vi "ConfigureAcquisition.vi"(8 "error in (no error)":errorcluster, 11 "NIScope in":refnum<class "NIScope.lvclass">) -> (0 "error out":errorcluster, 3 "NIScope out":refnum<class "NIScope.lvclass">)   [LabVIEW 2018, in "ScopePlugins.lvlib" / "NIScope.lvclass"]
doc: "This VI configures the horizontal settings."
uses:
  NIScope.lvclass
  C:/projects/ICDAS/NistPluggableModules/Scope/ScopePlugins/ScopePluginBaseClass/ScopePluginsBase.lvclass
  ScopePluginBaseClass/ScopePluginsBase.lvclass/ScopePluginsBase.ctl
  NIScope.lvclass/NIScope.ctl
  <instrlib>/niScope/Controls/niScope acquisition type.ctl
  ScopePluginBaseClass/Accessors/Write Channels.vi
  ScopePluginBaseClass/Accessors/Read Channels.vi
  <vilib>/Utility/error.llb/Error Cluster From Error Code.vi
  <vilib>/ErrorRing/Error Ring.xnode
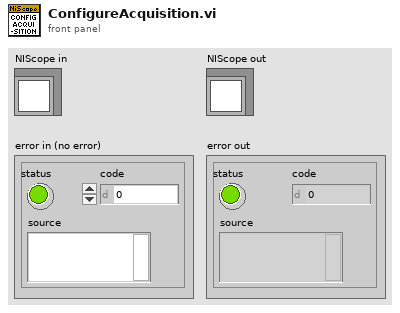
[diagram p1: front panel]
types:
  T1 = typedef "ScopePlugins.lvlib/ScopePluginsBase.lvclass/InitializationSettings.ctl" = cluster{"Reset":bool, "IdQuery":bool, "AutoConfig":bool, "Options String":string, "Synchronize":bool}
  T2 = typedef "ScopePlugins.lvlib/ScopePluginsBase.lvclass/ChannelSetting(s).ctl" = cluster{"Number of Channels":i32, "Channel(s)":cluster{"Enabled":bool, "Instrument Handle":string, "Channel Name":string, "Maximum Input Frequency":dbl, "Verticle Settings":cluster{"Vertical Range":dbl, "Vertical Offset":dbl, "Probe Attenuation":dbl, "Vertical Coupling":i32}, "Connected":bool, "Input Impedance":dbl, "IO Type Instrument Handle":refnum<k15>}[]}
  T3 = cluster{"Enabled":bool, "Instrument Handle":string, "Channel Name":string, "Maximum Input Frequency":dbl, "Verticle Settings":cluster{"Vertical Range":dbl, "Vertical Offset":dbl, "Probe Attenuation":dbl, "Vertical Coupling":i32}, "Connected":bool, "Input Impedance":dbl, "IO Type Instrument Handle":refnum<k15>}[]
  T4 = typedef "ScopePlugins.lvlib/ScopePluginsBase.lvclass/HorizontalSettings.ctl" = cluster{"Continuous":bool, "EnableAveraging":bool, "Number Averages":i32, "Measurement Timeout":dbl, "Min Record Length":i32, "Min Sample Rate":dbl, "Enforce Realtime":bool, "Sampling Mode ":enum16{"Real Time", "Equivalent Time", "Segment", "Real Time Peak Detect", "Real Time High Resolution", "Peak Detect Segment", "High Resolution Segment"}, "Interpolation":enum16{"No Interpolation", "sin(x)/x", "linear", "1 Point sin(x)/x", "2 Point sin(x)/x", "4 Point sin(x)/x", "8 Point sin(x)/x", "16 Point sin(x)/x"}, "Type":enum16{"Normal", "PeakDetect", "HighRes", "Envelope", "Average"}, "StartTime":dbl, "Time Per Record":dbl, "Number of Points Minimum":i32, "Measurement Name":string, "Measurement RefreshTime (ms)":u32}
  T5 = enum16{"Normal", "PeakDetect", "HighRes", "Envelope", "Average"}
  T6 = typedef "niScope acquisition type.ctl" = i32
  T7 = cluster{"Enabled":bool, "Instrument Handle":string, "Channel Name":string, "Maximum Input Frequency":dbl, "Verticle Settings":cluster{"Vertical Range":dbl, "Vertical Offset":dbl, "Probe Attenuation":dbl, "Vertical Coupling":i32}, "Connected":bool, "Input Impedance":dbl, "IO Type Instrument Handle":refnum<k15>}
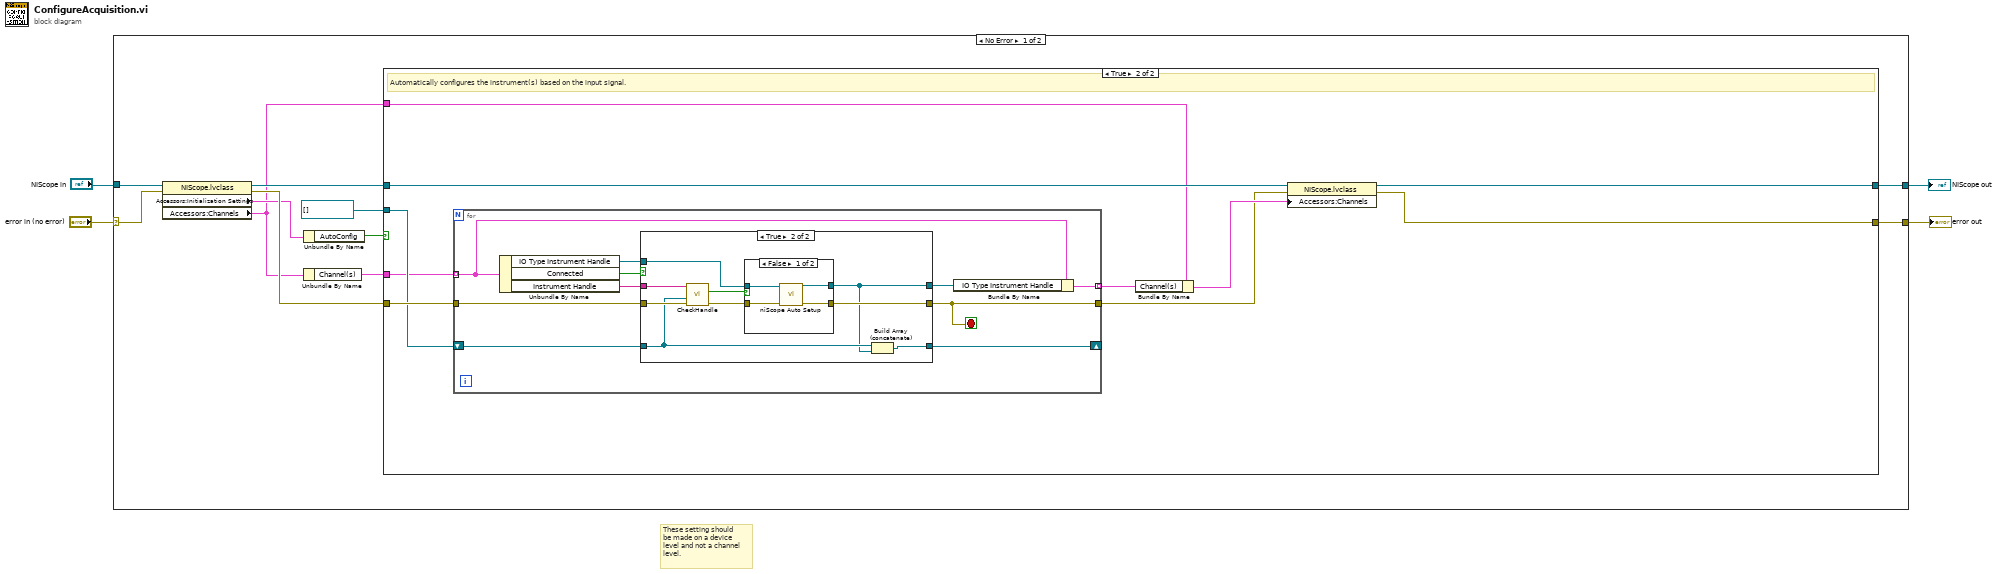
[diagram p0: block diagram]
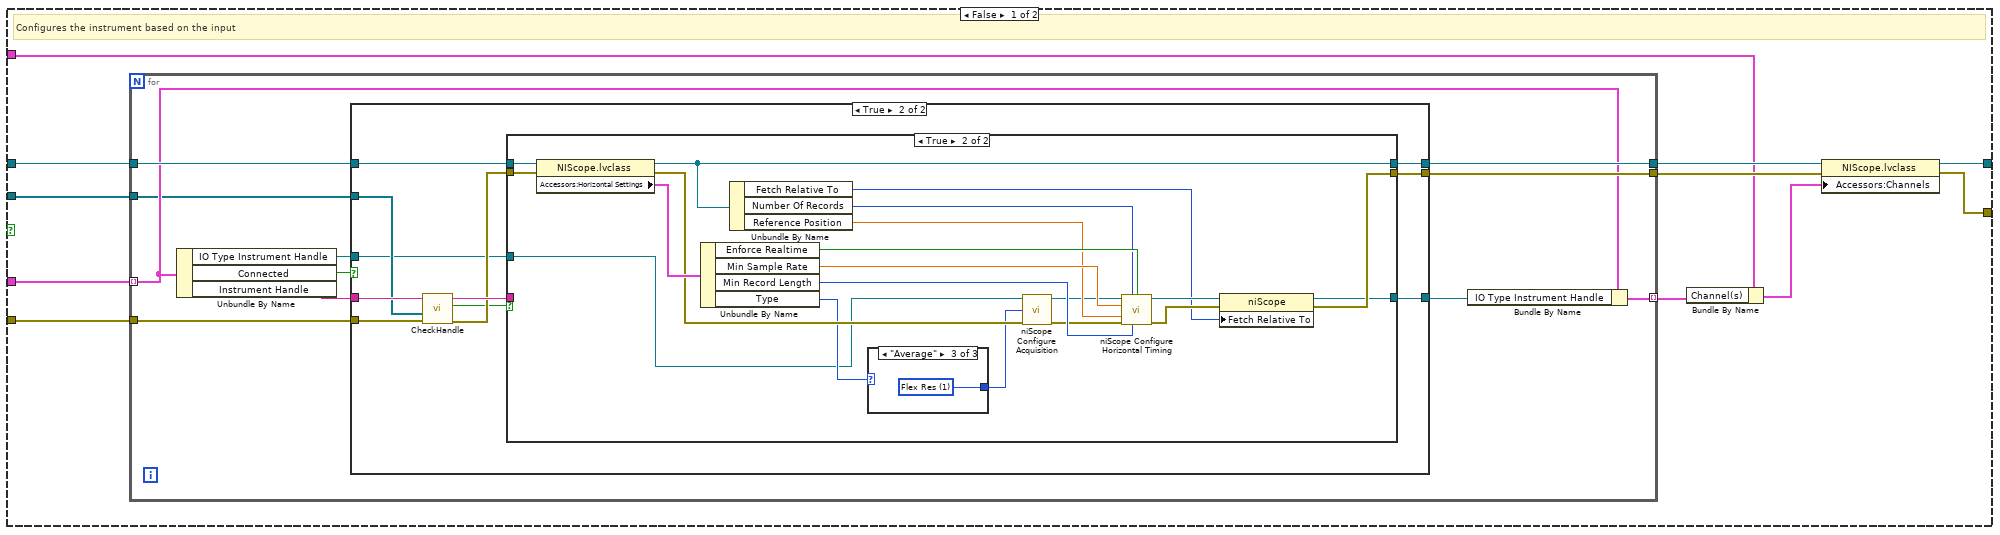
[diagram p2: hidden frame]
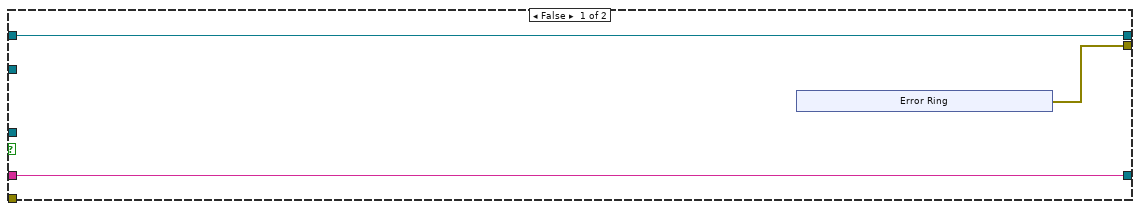
[diagram p3: hidden frame]
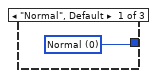
[diagram p5: hidden frame]
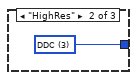
[diagram p6: hidden frame]
diagram:
  # "These setting should\nbe made on a device\nlevel and not a channel\nlevel."
  n1 = case shown="No Error" "error in (no error)" {
    selector: "error in (no error)" -> [w15 w121]
    tunnel: "NIScope in" -> [w14 w122]
    tunnel: [w10 w122] -> w2
    tunnel: [w9 w121] -> w1
    frame No Error {
      n2 = property class="NIScope.lvclass"(reference=w14, error in=w15) -> (reference out=w13:refnum<class "NIScope.lvclass">, error out=w12:errorcluster, "Accessors:Initialization Settings"=w6:T1, "Accessors:Channels"=w5:T2)
      n3 = Unbundle By Name(w6) -> ("AutoConfig"=w8:bool)
      n4 = Unbundle By Name(w5) -> ("Channel(s)"=w11:T3)
      n5 = case shown="True" w8 {
        tunnel: w13 -> [w25 w88]
        tunnel: w12 -> [w24 w92]
        tunnel: w11 -> [w17 w85]
        tunnel: [w23 w89] -> w10
        tunnel: [w21 w87] -> w9
        tunnel: refnum<k15>[] [] ("Array") -> [w18 w91]
        tunnel: w5 -> [w16 w83]
        frame False {
          # "Configures the instrument based on the input"
          n6 = for {
            tunnel: [w37] -> w26
            tunnel: w25 -> [w36]
            tunnel: w17 -> [w30] mode=indexing
            tunnel: [w31] -> w19 mode=indexing
            tunnel: w18 -> [w28]
            tunnel: w24 -> [w35]
            tunnel: [w33] -> w22
            n7 = Unbundle By Name(w30) -> ("IO Type Instrument Handle"=w27:refnum<k15>, "Connected"=w29:bool, "Instrument Handle"=w34:string)
            n8 = case shown="True" w29 {
              tunnel: w36 -> [w40 w56]
              tunnel: [w40 w55] -> w37
              tunnel: [w39 w53] -> w33
              tunnel: w35 -> [_ w49]
              tunnel: w34 -> [w38 w52]
              tunnel: [w38 w54] -> w32
              tunnel: w28 -> [_ w51]
              tunnel: w27 -> [_ w46]
              frame False {
                n9 = xnode "Error Ring"() -> ("error out"=w39:errorcluster)
              }
              frame True {
                n10 = call "CheckHandle.vi"("error in (no error)"=w49, "Array"=w51, "Handle In"=w52) -> ("error out"=w48:errorcluster, "Duplicate Instrument?"=w47:bool, "Handle Out"=w50:string)  [unwired: 6 in]
                n11 = case shown="True" w47 {
                  tunnel: w56 -> [w59 w79]
                  tunnel: [w59 w67] -> w55
                  tunnel: [w57 w74] -> w54
                  tunnel: [w58 w75] -> w53
                  tunnel: w50 -> [w57 _]
                  tunnel: w48 -> [w58 w78]
                  tunnel: w46 -> [_ w60]
                  frame False {
                  }
                  frame True {
                    n12 = property class="NIScope.lvclass"(reference=w79, error in=w78) -> (reference out=w67:refnum<class "NIScope.lvclass">, error out=w66:errorcluster, "Accessors:Horizontal Settings"=w73:T4)
                    n13 = Unbundle By Name(w73) -> ("Enforce Realtime"=w72:bool, "Min Sample Rate"=w71:dbl, "Min Record Length"=w68:i32, "Type"=w63:T5)
                    n14 = Unbundle By Name(w67) -> ("Fetch Relative To"=w61:i32, "Number Of Records"=w70:i32, "Reference Position"=w69:dbl)
                    n15 = case shown="\"Average\"" w63 {
                      tunnel: [w80 w81 w82] -> w62
                      frame "Normal", Default {
                        w80 = T6 0 items=["Normal"=0, "Flex Res"=1, "DDC"=3] ("acquisition Type")
                      }
                      frame "HighRes" {
                        w81 = T6 3 items=["Normal"=0, "Flex Res"=1, "DDC"=3] ("acquisition Type")
                      }
                      frame "Average" {
                        w82 = T6 1 items=["Normal"=0, "Flex Res"=1, "DDC"=3] ("acquisition Type")
                      }
                    }
                    n16 = call <instrlib>:"niScope Configure Acquisition.vi"("instrument handle"=w60, "acquisition Type"=w62, "error in"=w66) -> ("instrument handle out"=w64:refnum<k15>, "error out"=w65:errorcluster)  [unwired: 11 in]
                    n17 = call <instrlib>:"niScope Configure Horizontal Timing.vi"("instrument handle"=w64, "number of records"=w70, "enforce realtime"=w72, "min sample rate"=w71, "reference position"=w69, "error in"=w65, "min record length"=w68) -> ("instrument handle out"=w77:refnum<k15>, "error out"=w76:errorcluster)  [unwired: 7 in]
                    n18 = property on="Property Node" class="niScope"(reference=w77, error in=w76, "Fetch Relative To"=w61) -> (reference out=w74:refnum<k15>, error out=w75:errorcluster)
                  }
                }
              }
            }
            n19 = Bundle By Name(cluster=w30, "IO Type Instrument Handle"=w32) -> (w31:T7)
          }
          n20 = Bundle By Name(cluster=w16, "Channel(s)"=w19) -> (w20:T2)
          n21 = property class="NIScope.lvclass"(reference=w26, error in=w22, "Accessors:Channels"=w20) -> (reference out=w23:refnum<class "NIScope.lvclass">, error out=w21:errorcluster)
        }
        frame True {
          # "Automatically configures the instrument(s) based on the input signal."
          n22 = for {
            tunnel: w85 -> [w95] mode=indexing
            tunnel: w92 -> [w101]
            tunnel: [w102] -> w86
            shift-right: [w98] -> _
            shift-left: w91 -> [w99]
            tunnel: [w93] -> w84 mode=indexing
            stop <- w102 stop-if-true
            n23 = Unbundle By Name(w95) -> ("IO Type Instrument Handle"=w96:refnum<k15>, "Connected"=w97:bool, "Instrument Handle"=w100:string)
            n24 = case shown="True" w97 {
              tunnel: [w104 w114] -> w102
              tunnel: w101 -> [w104 w113]
              tunnel: w100 -> [_ w111]
              tunnel: w99 -> [w105 w109]
              tunnel: [w105 w108] -> w98
              tunnel: w96 -> [w103 w107]
              tunnel: [w103 w106] -> w94
              frame False {
              }
              frame True {
                n25 = call "CheckHandle.vi"("error in (no error)"=w113, "Array"=w109, "Handle In"=w111) -> ("error out"=w112:errorcluster, "Duplicate Instrument?"=w110:bool)  [unwired: 6 in, 1 out]
                n26 = case shown="False" w110 {
                  tunnel: w107 -> [w118 w119]
                  tunnel: w112 -> [w117 w120]
                  tunnel: [w116 w120] -> w114
                  tunnel: [w115 w119] -> w106
                  frame False {
                    n27 = call <instrlib>:"niScope Auto Setup.vi"("instrument handle"=w118, "error in"=w117) -> ("instrument handle out"=w115:refnum<k15>, "error out"=w116:errorcluster)  [unwired: 12 in]
                  }
                  frame True {
                  }
                }
                n28 = Build Array (concatenate)(w109, w106) -> (w108:refnum<k15>[])
              }
            }
            n29 = Bundle By Name(cluster=w95, "IO Type Instrument Handle"=w94) -> (w93:T7)
          }
          n30 = Bundle By Name(cluster=w83, "Channel(s)"=w84) -> (w90:T2)
          n31 = property class="NIScope.lvclass"(reference=w88, error in=w86, "Accessors:Channels"=w90) -> (reference out=w89:refnum<class "NIScope.lvclass">, error out=w87:errorcluster)
        }
      }
    }
    frame Error {
    }
  }
  "error out" <- w1
  "NIScope out" <- w2
